vi "TCP Write.vi"(0 "connection ID":refnum<k5>, 5 "data string":string, 9 "timeout (ms)":i32=5000, 11 "error in (no error)":errorcluster) -> (4 "connection ID out":refnum<k5>, 8 "bytes written":i32, 15 "error out":errorcluster)   [LabVIEW 2020]
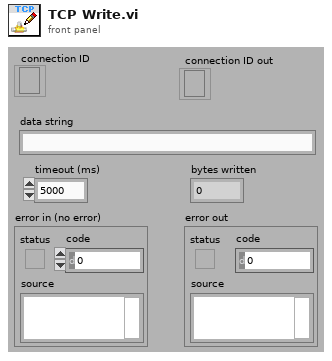
[diagram p1: front panel]
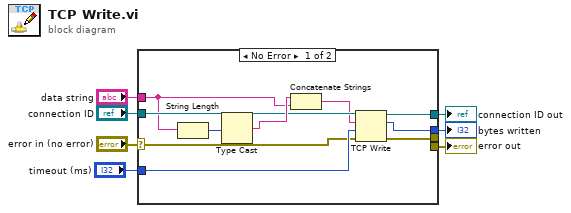
[diagram p0: block diagram]
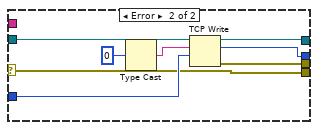
[diagram p2: hidden frame]
diagram:
  n1 = case shown="No Error" "error in (no error)" {
    selector: "error in (no error)" -> [w10 w19]
    tunnel: [w17 w19] -> w7
    tunnel: [w16 w24] -> w6
    tunnel: "connection ID" -> [w11 w25]
    tunnel: "timeout (ms)" -> [w14 w22]
    tunnel: [w12 w23] -> w3
    tunnel: "data string" -> [w9 _]
    tunnel: [_ w18] -> _
    frame No Error {
      n2 = String Length(string=w9) -> (length=w13:i32)
      n3 = Type Cast(x=w13) -> (*(type *) &x=w15:string)  [unwired: 1 in]
      n4 = Concatenate Strings(w15, w9) -> (w8:string)
      n5 = TCP Write(connection ID=w11, data in=w8, error in (no error)=w10, 9:w14) -> (connection ID out=w16:refnum<k5>, bytes written=w12:i32, error out=w17:errorcluster)
    }
    frame Error {
      n6 = Type Cast(x=0 ("bytes written")) -> (*(type *) &x=w21:string)  [unwired: 1 in]
      n7 = TCP Write(connection ID=w25, data in=w21, 9:w22) -> (connection ID out=w24:refnum<k5>, bytes written=w23:i32, error out=w18:errorcluster)  [unwired: 1 in]
    }
  }
  "error out" <- w7
  "bytes written" <- w3
  "connection ID out" <- w6
